vi "Hahn & RF with no RF ref Pulse Sequence Generator.vi"(0 "N Loop":i32=10000, 1 "Rabi Frequency":dbl, 2 "RF Pulse":dbl, 3 "Tau":dbl, 5 "AOM Pulse length":dbl=2.5e-06, 7 "AOM Rest time":dbl=1e-06, 9 "Signal Delay":dbl=6e-07, 11 "APD signal width":dbl=5e-07, 12 "MW Delay":dbl, 13 "Pulse offset":dbl) -> (4 "Pulse Sequence":T1(array[cluster]))   [LabVIEW 2012]
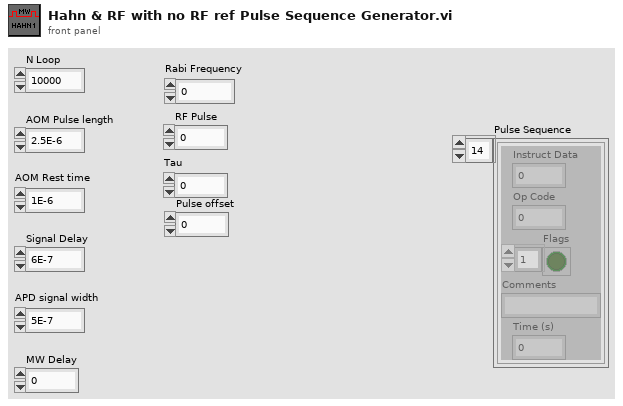
[diagram p1: front panel]
types:
  T1 = cluster{"Instruct Data":i32, "Op Code":i32, "Flags":bool[], "Comments":string, "Time (s)":dbl}[]
  T2 = cluster{"Instruct Data":i32, "Op Code":i32, "Flags":bool[], "Comments":string, "Time (s)":dbl}
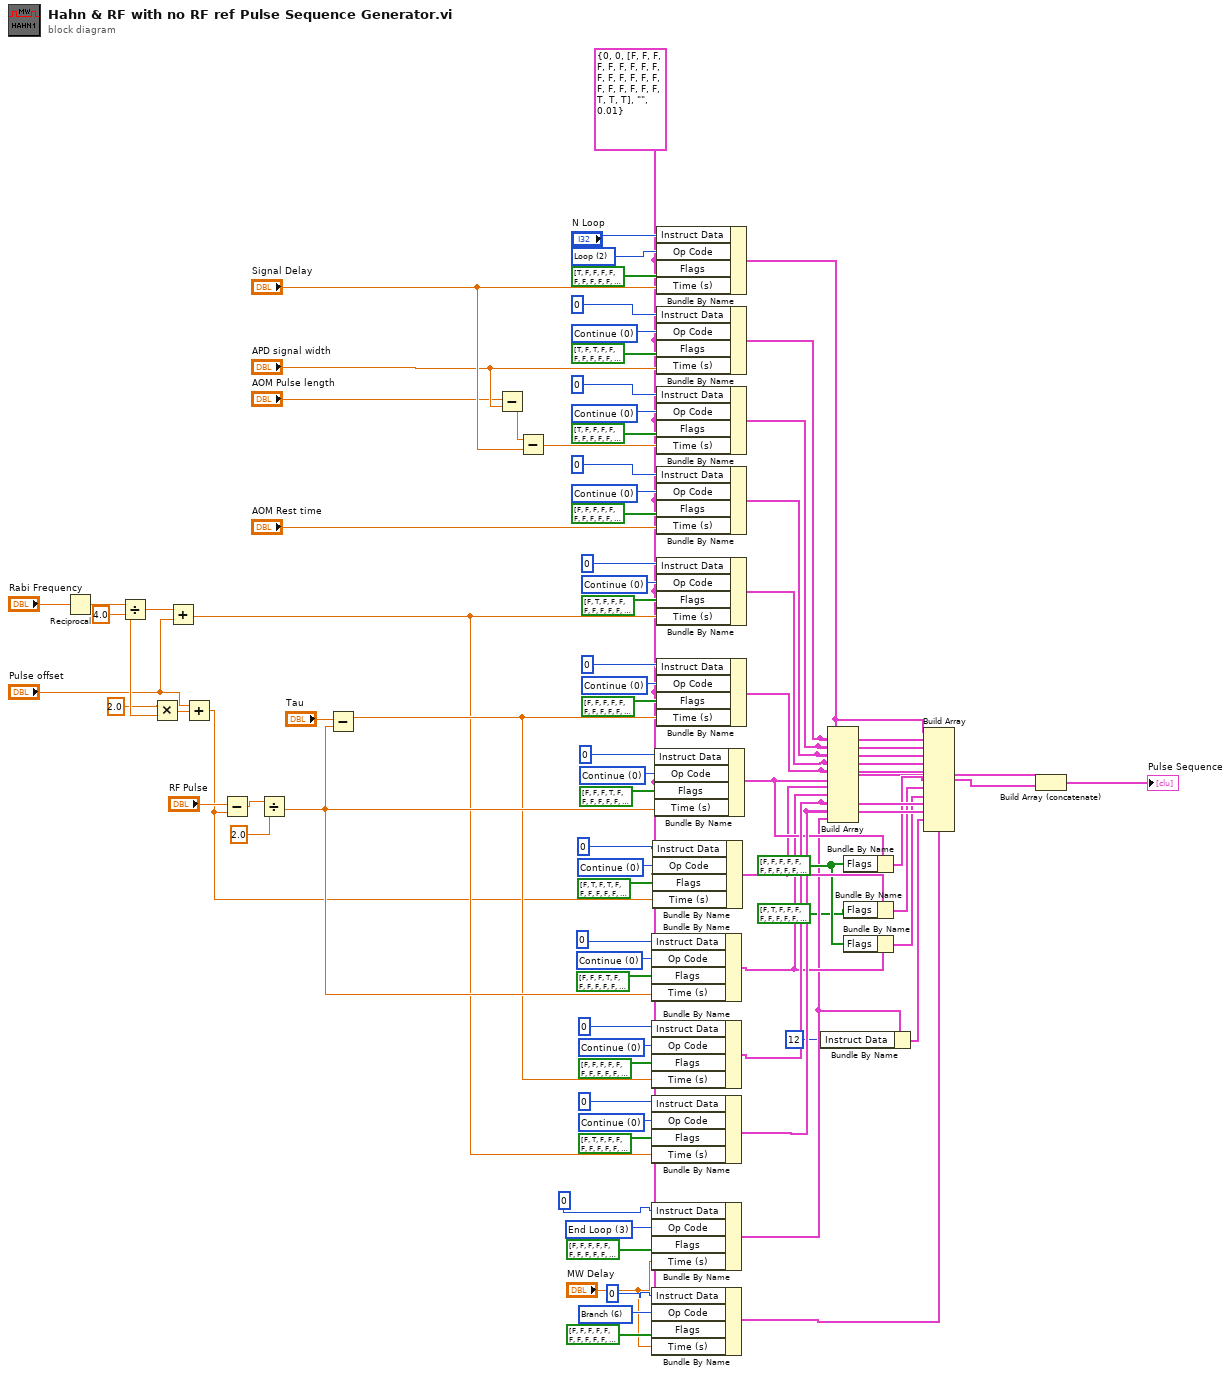
[diagram p0: block diagram]
diagram:
  w11 = bool[] [FALSE, FALSE, FALSE, FALSE, FALSE, FALSE, FALSE, FALSE, FALSE, FALSE, FALSE, FALSE, FALSE, FALSE, FALSE, FALSE, FALSE, FALSE, FALSE, FALSE, FALSE, TRUE, TRUE, TRUE] ("Flags")
  w27 = 6 items=["Continue", "Stop", "Loop", "End Loop", "JSR", "RTS", "Branch", "Long Delay", "Wait"] ("Op Code")
  w34 = 0 items=["Continue", "Stop", "Loop", "End Loop", "JSR", "RTS", "Branch", "Long Delay", "Wait"] ("Op Code")
  w37 = 0 items=["Continue", "Stop", "Loop", "End Loop", "JSR", "RTS", "Branch", "Long Delay", "Wait"] ("Op Code")
  w46 = 0 items=["Continue", "Stop", "Loop", "End Loop", "JSR", "RTS", "Branch", "Long Delay", "Wait"] ("Op Code")
  w49 = 0 items=["Continue", "Stop", "Loop", "End Loop", "JSR", "RTS", "Branch", "Long Delay", "Wait"] ("Op Code")
  w53 = 0 items=["Continue", "Stop", "Loop", "End Loop", "JSR", "RTS", "Branch", "Long Delay", "Wait"] ("Op Code")
  w56 = 0 items=["Continue", "Stop", "Loop", "End Loop", "JSR", "RTS", "Branch", "Long Delay", "Wait"] ("Op Code")
  w59 = 0 items=["Continue", "Stop", "Loop", "End Loop", "JSR", "RTS", "Branch", "Long Delay", "Wait"] ("Op Code")
  w66 = 3 items=["Continue", "Stop", "Loop", "End Loop", "JSR", "RTS", "Branch", "Long Delay", "Wait"] ("Op Code")
  w71 = 0 items=["Continue", "Stop", "Loop", "End Loop", "JSR", "RTS", "Branch", "Long Delay", "Wait"] ("Op Code")
  w75 = 0 items=["Continue", "Stop", "Loop", "End Loop", "JSR", "RTS", "Branch", "Long Delay", "Wait"] ("Op Code")
  w78 = 0 items=["Continue", "Stop", "Loop", "End Loop", "JSR", "RTS", "Branch", "Long Delay", "Wait"] ("Op Code")
  w80 = 2 items=["Continue", "Stop", "Loop", "End Loop", "JSR", "RTS", "Branch", "Long Delay", "Wait"] ("Op Code")
  w24 = T2 {"Instruct Data"=0, "Op Code"=0, "Flags"=[FALSE, FALSE, FALSE, FALSE, FALSE, FALSE, FALSE, FALSE, FALSE, FALSE, FALSE, FALSE, FALSE, FALSE, FALSE, FALSE, FALSE, FALSE, FALSE, FALSE, FALSE, TRUE, TRUE, TRUE], "Comments"="", "Time (s)"=0.01} ("PB Inst 2")
  n1 = Reciprocal(x="Rabi Frequency") -> (1/x=w64:dbl)
  n2 = Divide(x=w64, y=4.0) -> (x/y=w63:dbl)
  n3 = Multiply(x=2.0, y=w63) -> (x*y=w51:dbl)
  n4 = Add(x=w63, y="Pulse offset") -> (x+y=w30:dbl)
  n5 = Add(x="Pulse offset", y=w51) -> (x+y=w29:dbl)
  n6 = Subtract(x="RF Pulse", y=w29) -> (x-y=w42:dbl)
  n7 = Divide(x=w42, y=2.0) -> (x/y=w39:dbl)
  n8 = Subtract(x="Tau", y=w39) -> (x-y=w32:dbl)
  n9 = Subtract(x="AOM Pulse length", y="APD signal width") -> (x-y=w73:dbl)
  n10 = Subtract(x=w73, y="Signal Delay") -> (x-y=w69:dbl)
  n11 = Bundle By Name(cluster=w24, "Instruct Data"=0, "Op Code"=w46, "Flags"=bool[] [FALSE, FALSE, FALSE, TRUE, FALSE, FALSE, FALSE, FALSE, FALSE, FALSE, FALSE, FALSE, FALSE, FALSE, FALSE, FALSE, FALSE, FALSE, FALSE, FALSE, FALSE, TRUE, TRUE, TRUE], "Time (s)"=w39) -> (w12:T2)
  n12 = Bundle By Name(cluster=w24, "Instruct Data"=0, "Op Code"=w37, "Flags"=bool[] [FALSE, FALSE, FALSE, FALSE, FALSE, FALSE, FALSE, FALSE, FALSE, FALSE, FALSE, FALSE, FALSE, FALSE, FALSE, FALSE, FALSE, FALSE, FALSE, FALSE, FALSE, TRUE, TRUE, TRUE], "Time (s)"=w32) -> (w17:T2)
  n13 = Bundle By Name(cluster=w24, "Instruct Data"=0, "Op Code"=w34, "Flags"=bool[] [FALSE, TRUE, FALSE, FALSE, FALSE, FALSE, FALSE, FALSE, FALSE, FALSE, FALSE, FALSE, FALSE, FALSE, FALSE, FALSE, FALSE, FALSE, FALSE, FALSE, FALSE, TRUE, TRUE, TRUE], "Time (s)"=w30) -> (w16:T2)
  n14 = Bundle By Name(cluster=w24, "Instruct Data"=0 ("y"), "Op Code"=w66, "Flags"=bool[] [FALSE, FALSE, FALSE, FALSE, FALSE, FALSE, FALSE, FALSE, FALSE, FALSE, FALSE, FALSE, FALSE, FALSE, FALSE, FALSE, FALSE, FALSE, FALSE, FALSE, FALSE, TRUE, TRUE, TRUE], "Time (s)"="MW Delay") -> (w4:T2)
  n15 = Bundle By Name(cluster=w24, "Instruct Data"=0 ("y"), "Op Code"=w27, "Flags"=bool[] [FALSE, FALSE, FALSE, FALSE, FALSE, FALSE, FALSE, FALSE, FALSE, FALSE, FALSE, FALSE, FALSE, FALSE, FALSE, FALSE, FALSE, FALSE, FALSE, FALSE, FALSE, TRUE, TRUE, TRUE], "Time (s)"="MW Delay") -> (w15:T2)
  n16 = Bundle By Name(cluster=w24, "Instruct Data"=0, "Op Code"=w49, "Flags"=bool[] [FALSE, TRUE, FALSE, TRUE, FALSE, FALSE, FALSE, FALSE, FALSE, FALSE, FALSE, FALSE, FALSE, FALSE, FALSE, FALSE, FALSE, FALSE, FALSE, FALSE, FALSE, TRUE, TRUE, TRUE], "Time (s)"=w29) -> (w13:T2)
  n17 = Bundle By Name(cluster=w24, "Instruct Data"=0, "Op Code"=w53, "Flags"=bool[] [FALSE, FALSE, FALSE, TRUE, FALSE, FALSE, FALSE, FALSE, FALSE, FALSE, FALSE, FALSE, FALSE, FALSE, FALSE, FALSE, FALSE, FALSE, FALSE, FALSE, FALSE, TRUE, TRUE, TRUE], "Time (s)"=w39) -> (w14:T2)
  n18 = Bundle By Name(cluster=w24, "Instruct Data"="N Loop", "Op Code"=w80, "Flags"=bool[] [TRUE, FALSE, FALSE, FALSE, FALSE, FALSE, FALSE, FALSE, FALSE, FALSE, FALSE, FALSE, FALSE, FALSE, FALSE, FALSE, FALSE, FALSE, FALSE, FALSE, FALSE, TRUE, TRUE, TRUE], "Time (s)"="Signal Delay") -> (w23:T2)
  n19 = Bundle By Name(cluster=w24, "Instruct Data"=0, "Op Code"=w78, "Flags"=bool[] [TRUE, FALSE, TRUE, FALSE, FALSE, FALSE, FALSE, FALSE, FALSE, FALSE, FALSE, FALSE, FALSE, FALSE, FALSE, FALSE, FALSE, FALSE, FALSE, FALSE, FALSE, TRUE, TRUE, TRUE], "Time (s)"="APD signal width") -> (w22:T2)
  n20 = Bundle By Name(cluster=w24, "Instruct Data"=0, "Op Code"=w75, "Flags"=bool[] [TRUE, FALSE, FALSE, FALSE, FALSE, FALSE, FALSE, FALSE, FALSE, FALSE, FALSE, FALSE, FALSE, FALSE, FALSE, FALSE, FALSE, FALSE, FALSE, FALSE, FALSE, TRUE, TRUE, TRUE], "Time (s)"=w69) -> (w21:T2)
  n21 = Bundle By Name(cluster=w24, "Instruct Data"=0, "Op Code"=w71, "Flags"=bool[] [FALSE, FALSE, FALSE, FALSE, FALSE, FALSE, FALSE, FALSE, FALSE, FALSE, FALSE, FALSE, FALSE, FALSE, FALSE, FALSE, FALSE, FALSE, FALSE, FALSE, FALSE, TRUE, TRUE, TRUE], "Time (s)"="AOM Rest time") -> (w20:T2)
  n22 = Bundle By Name(cluster=w24, "Instruct Data"=0, "Op Code"=w59, "Flags"=bool[] [FALSE, TRUE, FALSE, FALSE, FALSE, FALSE, FALSE, FALSE, FALSE, FALSE, FALSE, FALSE, FALSE, FALSE, FALSE, FALSE, FALSE, FALSE, FALSE, FALSE, FALSE, TRUE, TRUE, TRUE], "Time (s)"=w30) -> (w19:T2)
  n23 = Bundle By Name(cluster=w24, "Instruct Data"=0, "Op Code"=w56, "Flags"=bool[] [FALSE, FALSE, FALSE, FALSE, FALSE, FALSE, FALSE, FALSE, FALSE, FALSE, FALSE, FALSE, FALSE, FALSE, FALSE, FALSE, FALSE, FALSE, FALSE, FALSE, FALSE, TRUE, TRUE, TRUE], "Time (s)"=w32) -> (w18:T2)
  n24 = Bundle By Name(cluster=w4, "Instruct Data"=12) -> (w2:T2)
  n25 = Build Array(w23, w22, w21, w20, w19, w18, w14, w13, w12, w17, w16, w4) -> (w7:T1)
  n26 = Bundle By Name(cluster=w14, "Flags"=w11) -> (w10:T2)
  n27 = Bundle By Name(cluster=w13, "Flags"=bool[] [FALSE, TRUE, FALSE, FALSE, FALSE, FALSE, FALSE, FALSE, FALSE, FALSE, FALSE, FALSE, FALSE, FALSE, FALSE, FALSE, FALSE, FALSE, FALSE, FALSE, FALSE, TRUE, TRUE, TRUE]) -> (w9:T2)
  n28 = Bundle By Name(cluster=w12, "Flags"=w11) -> (w8:T2)
  n29 = Build Array(w23, w22, w21, w20, w19, w18, w10, w9, w8, w17, w16, w2, w15) -> (w6:T1)
  n30 = Build Array (concatenate)(w7, w6) -> (→"Pulse Sequence":T1)
